vi "ROI grp-Delete selected ROIs from table.vi"(8 "error in (no error)":errorcluster, 11 "Table in":refnum<vi>) -> (0 "error out":errorcluster, 2 "ROI number of ROIs deleted from each group.":T1(array[cluster]), 3 "Table out":refnum<vi>)   [LabVIEW 2020]
panel:
  out "Deleted section":string[][](array[string])
  out "New value":string[][](array[string])
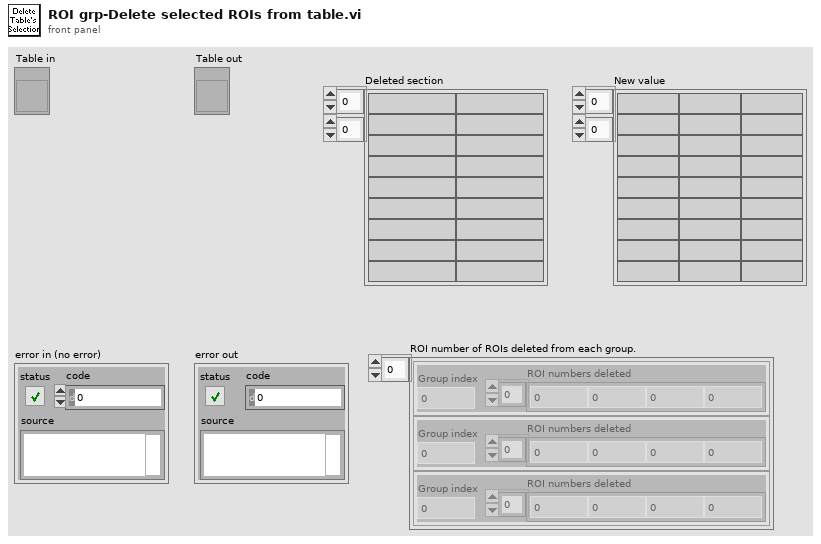
[diagram p1: front panel]
types:
  T1 = cluster{"Group index":i32, "ROI numbers deleted":i32[]}[]
  T2 = typedef "LVRowAndColumnTypeDef.ctl" = cluster{"Row":i32, "Column":i32}
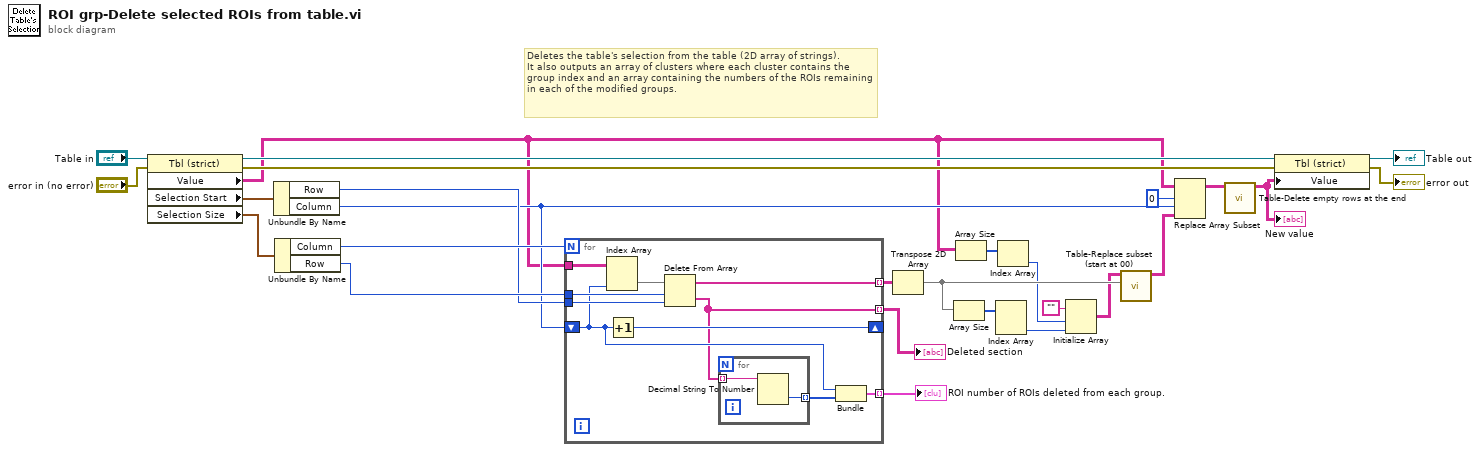
[diagram p0: block diagram]
diagram:
  # "Deletes the table's selection from the table (2D array of strings).\nIt also outputs an array of clusters where each cluster contains the group index and an array containing the numbers of the ROIs remaining in each of the modified groups."
  n1 = property on="Property Node" class="Tbl (strict)"(reference="Table in", error in="error in (no error)") -> (reference out=w22:refnum<vi>, error out=w27:errorcluster, "Value"=w4:string[][], "Selection Start"=w25:T2, "Selection Size"=w24:T2)
  n2 = Unbundle By Name(w25) -> ("Row"=w19:i32, "Column"=w18:i32)
  n3 = Unbundle By Name(w24) -> ("Column"=w23:i32, "Row"=w21:i32)
  n4 = for {
    N: w23 -> [_]
    tunnel: w4 -> [w37]
    shift-right: [w33] -> _
    shift-left: w18 -> [w30]
    tunnel: w19 -> [w35]
    tunnel: w21 -> [w34]
    tunnel: [w29] -> w20 mode=indexing
    tunnel: [w28] -> w1 mode=indexing
    tunnel: [w31] -> w2 mode=indexing
    n5 = Index Array "Index Array"(array=w37, index (col)=w30) -> (element=w36:string[])  [unwired: 1 in]
    n6 = Increment(x=w30) -> (x+1=w33:i32)
    n7 = Delete From Array "Delete From Array"(array=w36, length=w34, index=w35) -> (deleted portion=w28:string[], array with subset deleted=w29:string[])
    n8 = for {
      tunnel: w28 -> [w39] mode=indexing
      tunnel: [w38] -> w32 mode=indexing
      n9 = Decimal String To Number(string=w39) -> (number=w38:i32)  [unwired: 2 in, 1 out]
    }
    n10 = Bundle("Column"=w30, w32) -> (w31:cluster{"Column":i32, i32[]})  [unwired: 1 in]
  }
  "Deleted section" <- w1
  "ROI number of ROIs deleted from each group." <- w2
  n11 = Transpose 2D Array(2D array=w20) -> (transposed array=w13:string[][])
  n12 = Array Size(array=w13) -> (size(s)=w15:i32[])
  n13 = Array Size(array=w4) -> (size(s)=w14:i32[])
  n14 = Index Array(array=w15) -> (element #2=w11:i32)  [unwired: 2 in, 1 out]
  n15 = Index Array(array=w14) -> (element=w10:i32)  [unwired: 1 in]
  n16 = Initialize Array("", w10, w11) -> (w12:string[][])
  n17 = call <userlib>:"Table-Replace subset (start at 00).vi"("Table to replace with"=w13, "Original table"=w12) -> ("Table out"=w9:string[][])  [unwired: 8 in, 1 out]
  n18 = Replace Array Subset(array=w4, new element=w9, index (row)=0 ("disabled index (row)"), index (col)=w18) -> (w8:string[][])
  n19 = call <userlib>:"Table-Delete empty rows at the end.vi"("Value in"=w8) -> ("Value out"=w3:string[][])  [unwired: 10 in]
  "New value" <- w3
  n20 = property on="Property Node" class="Tbl (strict)"(reference=w22, error in=w27, "Value"=w3) -> (reference out=→"Table out":refnum<vi>, error out=→"error out":errorcluster)
